vi "frequency_aproximate.vi"() -> ()   [LabVIEW 2017]
panel:
  out "error IO":errorcluster
  out "y value":dbl
  in  "freq":dbl
  in  "Array":dbl[][](array[numeric])
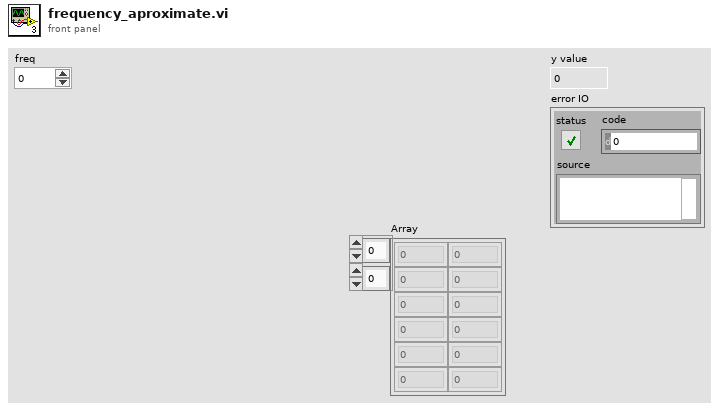
[diagram p1: front panel]
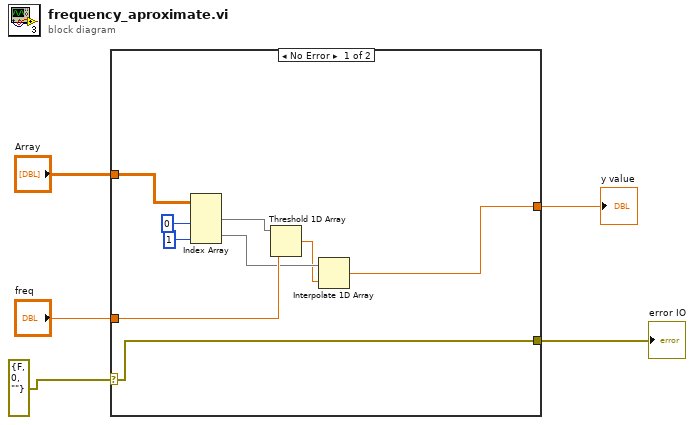
[diagram p0: block diagram]
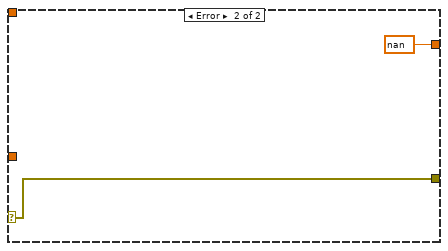
[diagram p2: hidden frame]
diagram:
  n1 = case shown="No Error" errorcluster {"status"=FALSE, "code"=0, "source"=""} ("error constant") {
    selector: errorcluster {"status"=FALSE, "code"=0, "source"=""} ("error constant") -> [w6 w16]
    tunnel: "Array" -> [w14 _]
    tunnel: "freq" -> [w11 _]
    tunnel: [w7 nan] -> w3
    tunnel: [w6 w16] -> w1
    frame No Error {
      n2 = Index Array(array=w14, index (col) #1=0 ("disabled index (col)"), index (col) #2=1 ("index (col)")) -> (element #1=w12:dbl[], element #2=w9:dbl[])  [unwired: 2 in]
      n3 = Threshold 1D Array(2:w11, 3:w12) -> (0:w8:dbl)  [unwired: 1 in]
      n4 = Interpolate 1D Array(1:w8, 2:w9) -> (0:w7:dbl)
    }
    frame Error {
    }
  }
  "y value" <- w3
  "error IO" <- w1
